vi "BRig_RT__Case_Exp__recordAnalogInput__PortC__netshar__v2.vi"(0 "input_buffer_dataAnalog":u16[][](array[numeric]), 1 "input_index":i32, 2 "input_iOccurence":u16, 3 "resetOccurrence":bool, 4 "input_dataCurrent":u16[](array[numeric]), 5 "input_empytyArray":u16[](array[numeric]), 6 "input_iState_start":T1, 8 "input_iState_end":T1, 10 "input_AI1":i16, 12 "input_AI0":i16) -> (13 "error out":errorcluster, 14 "output_buffer_dataAnalog":u16[][](array[numeric]), 15 "output_index":i32, 16 "output_iOccurrence":u16)   [LabVIEW 2014]
uses:
  myRIO_BRig_RT__Case_Exp_stateList.ctl
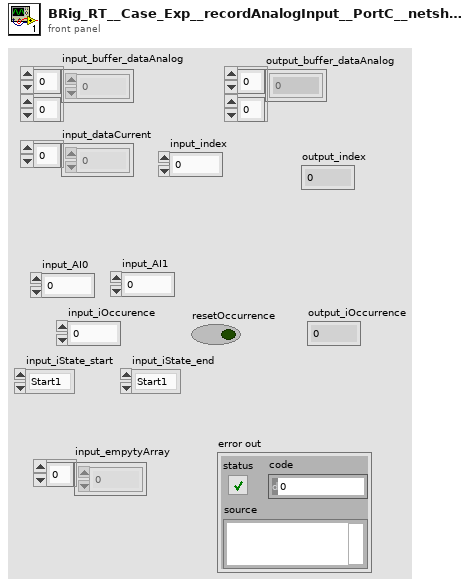
[diagram p1: front panel]
types:
  T1 = typedef "myRIO_BRig_RT__Case_Exp_stateList.ctl" = enum16{"Start1", "Start2", "Start3", "saveSettings1", "saveSettings2", "saveSettings3", "saveSettings4", "saveSettings_LC_ENL_l1", "saveSettings_LC_ENL_l2", "saveSettings_LC_Cue_l1", "saveSettings_LC_Cue_l2", "saveSettings6_LC_l1_Other", "SaveSettings6_LC_l2_Other", "setSettings_Audio", "setSettings_Laser", "initBlock_pre", "initBlock", "initBlock2", "initBlock_post", "initTrial_pre", "initTrial", "initTrial2", "initTrial3", "initTrial4", "initTrial_LC_ENL1", "initTrial_LC_Cue1", "initTrial_LC_Cue1_2", "initTrial_LC_Sel", "initTrial_post", "ENL1_pre", "ENL1", "ENL1_post", "ENL1Penalty_pre", "ENL1Penalty", "ENL2_pre", "ENL2", "ENL2Penalty_pre", "ENL2Penalty", "Cue1_pre", "Cue1", "Cue1_post", "Cue1Penalty_pre", "Cue1Penalty", "Cue2_pre", "Cue2", "Cue2Penalty_pre", "Cue2Penalty", "Selection_pre", "Selection", "Select_post", "SelectReward_pre", "SelectReward", "SelectRewardPost_pre", "SelectRewardPost", "SelectWrong_pre", "SelectWrong", "SelectWrong_post", "SelectTimeout_pre", "SelectTimeout", "SelectTimeout_post", "endTrial_pre", "endTrial1", "endTrial2", "endTrial3", "endTrial_post", "endBlock_pre", "endBlock", "endBlock_post", "endExp", "commConnect", "commUpload_pre", "commUpload_dataBlock", "commUpload_dataCurrent", "commUpload_dataExp", "commUpload_dataLC", "commUpload_dataTrial", "commUpload_post", "saveData_pre", "saveData_dataBlock", "saveData_dataCurrent", "saveData_dataExp", "saveData_dataLC", "saveData_dataTrial", "saveData_post", "empty_endBlock1", "empty_endBlock2", "empty_endTrial1", "empty_endTrial2", "empty_endTrial3", "empty_endTrial4", "empty_endTrial5", "dummyState", "dummyState_endBlock", "FreeReward_pre", "FreeReward", "FreeRewardPost_pre", "FreeRewardPost"}
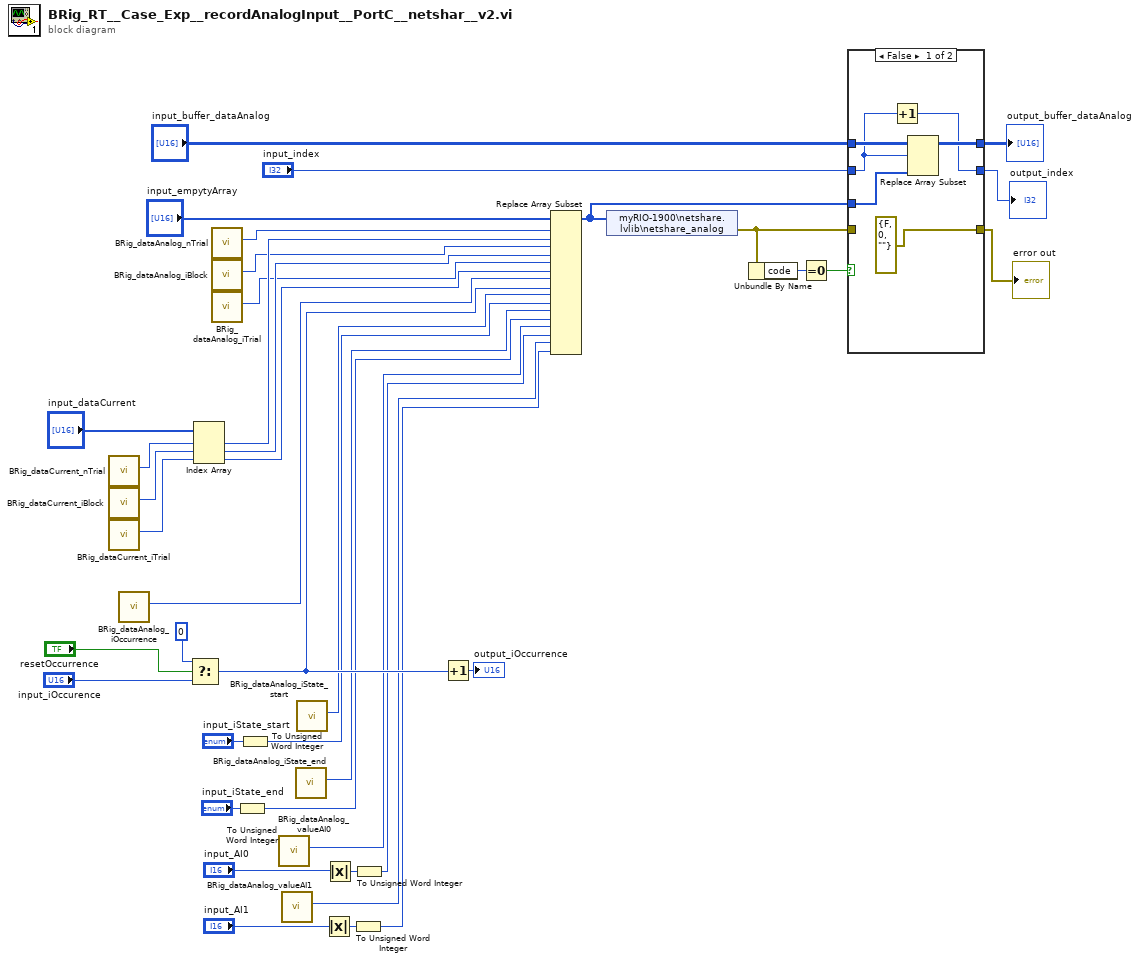
[diagram p0: block diagram]
diagram:
  n1 = call "BRig_dataCurrent_nTrial.vi"() -> ("output_nTrial"=w37:i32)  [unwired: 11 in]
  n2 = call "BRig_dataCurrent_iBlock.vi"() -> ("output_iBlock"=w36:i32)  [unwired: 11 in]
  n3 = call "BRig_dataCurrent_iTrial.vi"() -> ("output_iTrial"=w35:i32)  [unwired: 11 in]
  n4 = call "BRig_dataAnalog_iOccurrence.vi"() -> ("output_iOccurrence"=w18:i32)  [unwired: 11 in]
  n5 = Select(t=u16 0, s="resetOccurrence", f="input_iOccurence") -> (s? t:f=w17:u16)
  n6 = Index Array(array="input_dataCurrent", index #1=w37, index #2=w36, index #3=w35) -> (element #1=w23:u16, element #2=w21:u16, element #3=w19:u16)
  n7 = call "BRig_dataAnalog_nTrial.vi"() -> ("output_nTrial"=w24:i32)  [unwired: 11 in]
  n8 = call "BRig_dataAnalog_iBlock.vi"() -> ("output_iBlock"=w22:i32)  [unwired: 11 in]
  n9 = call "BRig_dataAnalog_iTrial.vi"() -> ("output_iTrial"=w20:i32)  [unwired: 11 in]
  n10 = To Unsigned Word Integer(number="input_iState_end") -> (unsigned 16bit integer=w13:u16)
  n11 = To Unsigned Word Integer(number="input_iState_start") -> (unsigned 16bit integer=w15:u16)
  n12 = call "BRig_dataAnalog_valueAI0.vi"() -> ("output_valueAI0"=w12:i32)  [unwired: 11 in]
  n13 = call "BRig_dataAnalog_valueAI1.vi"() -> ("output_valueAI1"=w10:i32)  [unwired: 11 in]
  n14 = call "BRig_dataAnalog_iState_end.vi"() -> ("output_iState_end"=w14:i32)  [unwired: 11 in]
  n15 = call "BRig_dataAnalog_iState_start.vi"() -> ("output_iState_start"=w16:i32)  [unwired: 11 in]
  n16 = Absolute Value(x="input_AI1") -> (abs(x)=w39:i16)
  n17 = Absolute Value(x="input_AI0") -> (abs(x)=w40:i16)
  n18 = To Unsigned Word Integer(number=w39) -> (unsigned 16bit integer=w9:u16)
  n19 = To Unsigned Word Integer(number=w40) -> (unsigned 16bit integer=w11:u16)
  n20 = Increment(x=w17) -> (x+1=→"output_iOccurrence":u16)
  n21 = Replace Array Subset(array="input_empytyArray", new element #1=w23, index #1=w24, new element #2=w21, index #2=w22, new element #3=w19, index #3=w20, new element #4=w17, index #4=w18, new element #5=w15, index #5=w16, new element #6=w13, index #6=w14, new element #7=w11, index #7=w12, new element #8=w9, index #8=w10) -> (w4:u16[])
  n22 = shared-variable "myRIO-1900\\netshare.lvlib\\netshare_analog"(w4) -> (error out=w3:errorcluster)  [unwired: 1 in]
  n23 = Unbundle By Name(w3) -> ("code"=w26:i32)
  n24 = Equal To 0?(x=w26) -> (x = 0?=w8:bool)
  n25 = case shown="False" w8 {
    tunnel: "input_buffer_dataAnalog" -> [w46 w49]
    tunnel: "input_index" -> [w43 w48]
    tunnel: [w45 w49] -> w6
    tunnel: [w42 w48] -> w5
    tunnel: w4 -> [w44 _]
    tunnel: w3 -> [_ w47]
    tunnel: [errorcluster {"status"=FALSE, "code"=0, "source"=""} ("error out") w47] -> w2
    frame False {
      n26 = Increment(x=w43) -> (x+1=w42:i32)
      n27 = Replace Array Subset(array=w46, new element=w44, index (row)=w43) -> (w45:u16[][])  [unwired: 1 in]
    }
    frame True {
    }
  }
  "output_buffer_dataAnalog" <- w6
  "output_index" <- w5
  "error out" <- w2
